vi "Toggle.vi"(8 "Error In":errorcluster, 11 "Tree Control In":refnum<vi>) -> (0 "Error Out":errorcluster, 3 "Tree Control Out":refnum<vi>)   [LabVIEW 2018, in "TraceTreeEditor.lvlib"]
uses:
  TraceTreeEditor.lvlib
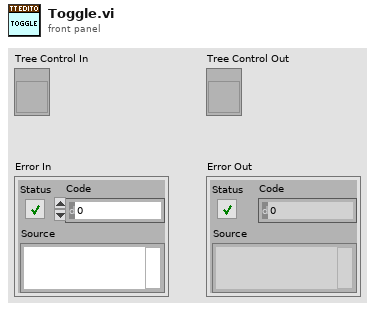
[diagram p1: front panel]
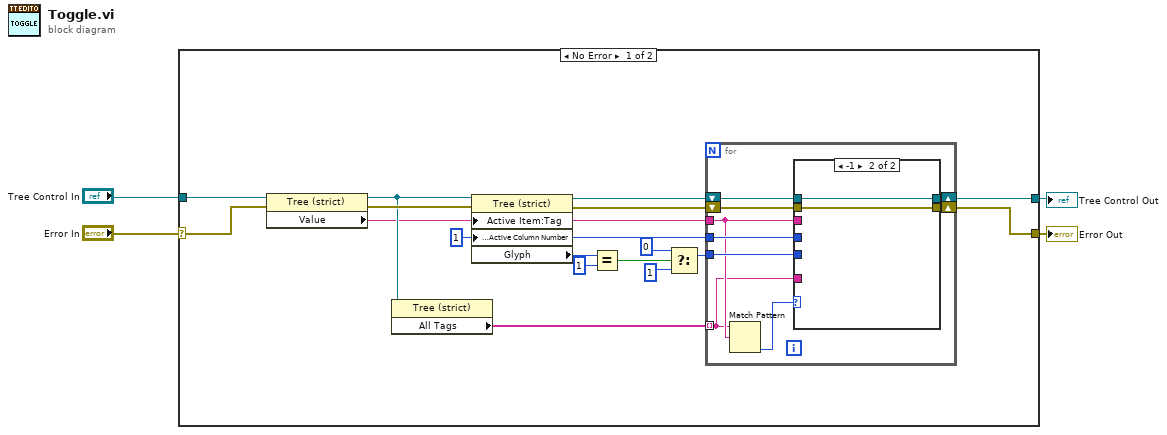
[diagram p0: block diagram]
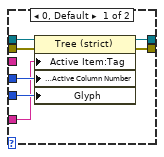
[diagram p2: hidden frame]
diagram:
  n1 = case shown="No Error" "Error In" {
    selector: "Error In" -> [w21 w40]
    tunnel: [w15 _] -> w2
    tunnel: "Tree Control In" -> [w5 _]
    tunnel: [w18 w40] -> w3
    frame No Error {
      w7 = 1 ("Active Cell:Active Column Number")
      n2 = property class="Tree (strict)"(reference=w5, error in=w21) -> (reference out=w17:refnum<vi>, error out=w20:errorcluster, "Value"=w11:string)
      n3 = property class="Tree (strict)"(reference=w17) -> ("All Tags"=w16:string[])  [unwired: 1 in, 2 out]
      n4 = property class="Tree (strict)"(reference=w17, error in=w20, "Active Item:Tag"=w11, "Active Cell:Active Column Number"=w7) -> (reference out=w6:refnum<vi>, error out=w19:errorcluster, "Glyph"=w8:i32)
      n5 = Equal?(x=w8, y=1) -> (x = y?=w10:bool)
      n6 = Select(t=0 ("y"), s=w10, f=1 ("y")) -> (s? t:f=w9:i32)
      n7 = for {
        tunnel: w7 -> [w27]
        tunnel: w9 -> [w26]
        tunnel: w11 -> [w24]
        shift-right: [w25] -> w15
        shift-left: w6 -> [w28]
        tunnel: w16 -> [w22] mode=indexing
        shift-right: [w29] -> w18
        shift-left: w19 -> [w30]
        n8 = Match Pattern(string=w22, regular expression=w24) -> (offset past match=w23:i32)  [unwired: 1 in, 3 out]
        n9 = case shown="-1" w23 {
          tunnel: w28 -> [w35 w38]
          tunnel: w27 -> [w34 _]
          tunnel: w26 -> [w33 _]
          tunnel: w24 -> [_ _]
          tunnel: [w32 w38] -> w25
          tunnel: w22 -> [w31 _]
          tunnel: w30 -> [w37 w39]
          tunnel: [w36 w39] -> w29
          frame 0, Default {
            n10 = property class="Tree (strict)"(reference=w35, error in=w37, "Active Item:Tag"=w31, "Active Cell:Active Column Number"=w34, "Glyph"=w33) -> (reference out=w32:refnum<vi>, error out=w36:errorcluster)
          }
          frame -1 {
          }
        }
      }
    }
    frame Error {
    }
  }
  "Tree Control Out" <- w2
  "Error Out" <- w3
